vi "Stop Core.vi"(10 "final error code":i32, 11 "First Actor in":refnum<class "First Actor.lvclass">) -> (3 "First Actor out":refnum<class "First Actor.lvclass">)   [LabVIEW 2021, in "First Actor.lvlib" / "First Actor.lvclass"]
doc: "(<B>Filename</B>: Actor Framework.lvlib:Actor.lvclass:Stop Core.vi)\n\nDefines what the actor does before it stops. Use the <B>final error code</B> input to determine whether the actor shut down in response to an error.\n\nBy default, this method passes the Stop message along to all auto-stop nested actors. A descendant class may override this method to define additional behavior, such as shutting down any processes the actor initiated in its override of the Actor Core method."
uses:
  First Actor.lvclass
  <vilib>/ActorFramework/Actor/Actor.lvclass
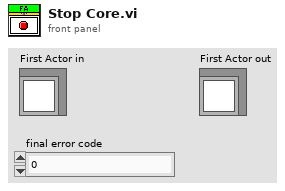
[diagram p1: front panel]
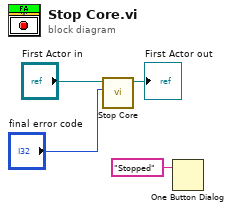
[diagram p0: block diagram]
diagram:
  n1 = call-parent "Stop Core.vi"("final error code"="final error code", "Actor in"="First Actor in") -> ("Actor out"=→"First Actor out":refnum<class "First Actor.lvclass">)  [unwired: 9 in]
  n2 = One Button Dialog(message="Stopped") -> ()  [unwired: 1 in, 1 out]
